vi "_PC_RTFunc_AccessSigRemrk.vi"(7 "Function":enum16{"Write", "Read"}(ring)=enum."Read", 8 "error in (no error)":errorcluster, 9 "Var in":variant) -> (0 "error out":errorcluster, 1 "Var out":variant)   [LabVIEW 2018]
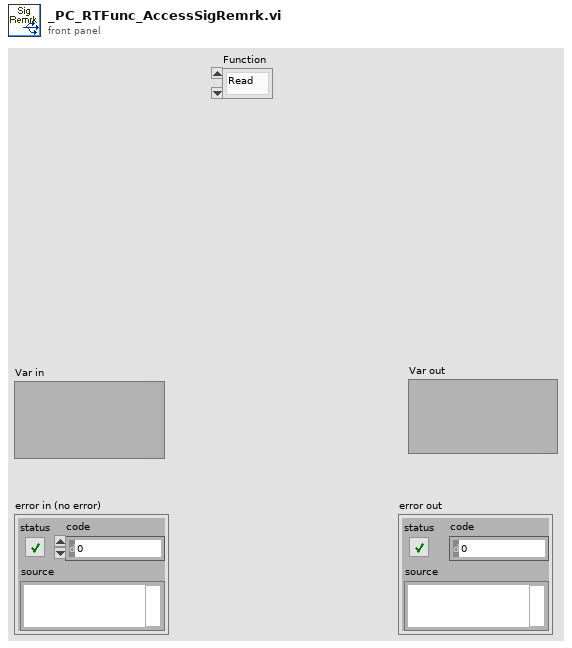
[diagram p1: front panel]
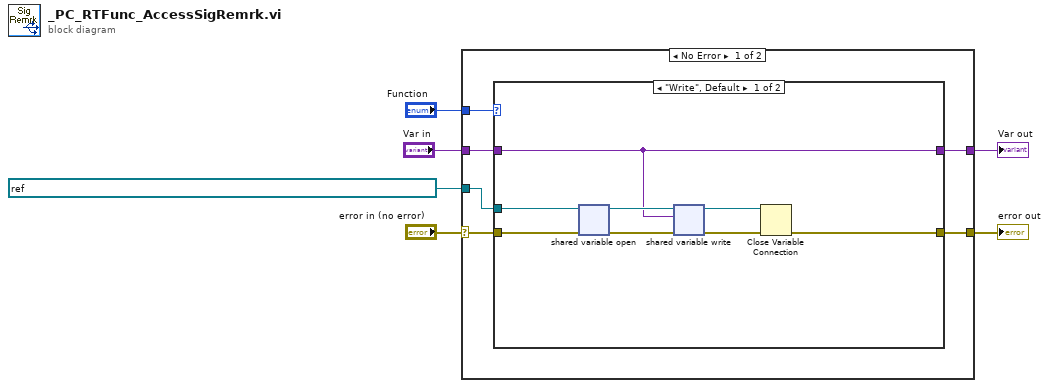
[diagram p0: block diagram]
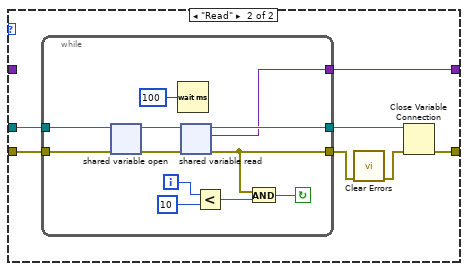
[diagram p2: hidden frame]
diagram:
  n1 = case shown="No Error" "error in (no error)" {
    selector: "error in (no error)" -> [w9 w41]
    tunnel: refnum<k21> "ni.var.psp://NI-sbRIO/_RT_CtrlLoop_WfmData_Variable/Wfm_SigRemrk" ("shared variable refnum in") -> [w12 _]
    tunnel: "Function" -> [w11 _]
    tunnel: [w10 w41] -> w4
    tunnel: [w7 w40] -> w3
    tunnel: "Var in" -> [w8 w40]
    frame No Error {
      n2 = case shown="\"Write\", Default" w11 {
        tunnel: w12 -> [w20 w27]
        tunnel: [w14 w25] -> w10
        tunnel: w9 -> [w19 w22]
        tunnel: [w13 w21] -> w7
        tunnel: w8 -> [w13 _]
        frame "Write", Default {
          n3 = shared-variable-open(w20, w19) -> (w18:refnum<k21>, w17:errorcluster)
          n4 = shared-variable-write(w18, w17, w13) -> (w16:refnum<k21>, w15:errorcluster)
          n5 = Close Variable Connection(8:w15, 11:w16) -> (0:w14:errorcluster)
        }
        frame "Read" {
          n6 = while {
            tunnel: w27 -> [w39]
            tunnel: [w37] -> w26
            tunnel: [w35] -> w21
            tunnel: [w29] -> w24
            tunnel: w22 -> [w28]
            i -> [w32]
            stop <- w30 continue-if-true
            n7 = shared-variable-open(w39, w28) -> (w38:refnum<k21>, w36:errorcluster)
            n8 = Wait (ms)(milliseconds to wait=u32 100) -> ()  [unwired: 1 out]
            n9 = shared-variable-read(w38, w36) -> (w37:refnum<k21>, w29:errorcluster, w35:variant)
            n10 = Less?(x=w32, y=10) -> (x < y?=w31:bool)
            n11 = And(x=w29, y=w31) -> (x .and. y?=w30:bool)
          }
          n12 = call <vilib>:"Clear Errors.vi"("error in (no error)"=w24) -> ("error out"=w23:errorcluster)  [unwired: 5 in, 1 out]
          n13 = Close Variable Connection(8:w23, 11:w26) -> (0:w25:errorcluster)
        }
      }
    }
    frame Error {
    }
  }
  "error out" <- w4
  "Var out" <- w3
